vi "Disconnect.vi"(8 "error in (no error)":errorcluster, 11 "midi out":refnum<class "midi out.lvclass">) -> (0 "error out":errorcluster)   [LabVIEW 2020, in "MIDIllan.lvlib" / "midi out.lvclass"]
doc: "Destroys a MIDI manager instance and releases its resources."
uses:
  midi out.lvclass
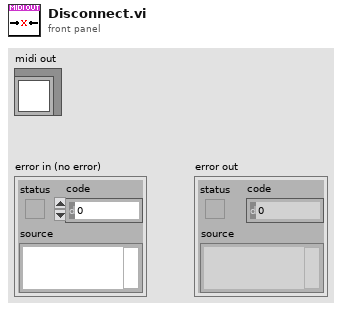
[diagram p1: front panel]
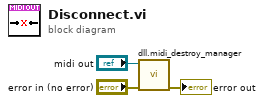
[diagram p0: block diagram]
diagram:
  n1 = call "dll.midi_destroy_manager.vi"("error in (no error)"="error in (no error)", "midi out in"="midi out") -> ("error out"=→"error out":errorcluster)  [unwired: 8 in, 1 out]
